vi "首页.vi"() -> ()   [LabVIEW 2016]
uses:
  <vilib>/Utility/miscctls.llb/LVPointTypeDef.ctl
  <vilib>/Utility/sysdir.llb/System Directory Type.ctl
  <vilib>/addons/database/_DB Variant To Data/Database Variant To Data.xnode
  PLC/PLC.lvlib
panel:
  out "大项目框 12":T1(xcontrol)
  out "大项目框 11":T1(xcontrol)
  out "大项目框 10":T1(xcontrol)
  out "大项目框 9":T1(xcontrol)
  out "大项目框 8":T1(xcontrol)
  out "大项目框 7":T1(xcontrol)
  out "大项目框 6":T1(xcontrol)
  out "大项目框 5":T1(xcontrol)
  out "大项目框 4":T1(xcontrol)
  out "大项目框 3":T1(xcontrol)
  out "大项目框 2":T1(xcontrol)
  out "大项目框":T1(xcontrol)
  out "湿度":string="75.5 %"
  out "室温":string="25.8 ℃"
  # "室温:"
  # "湿度:"
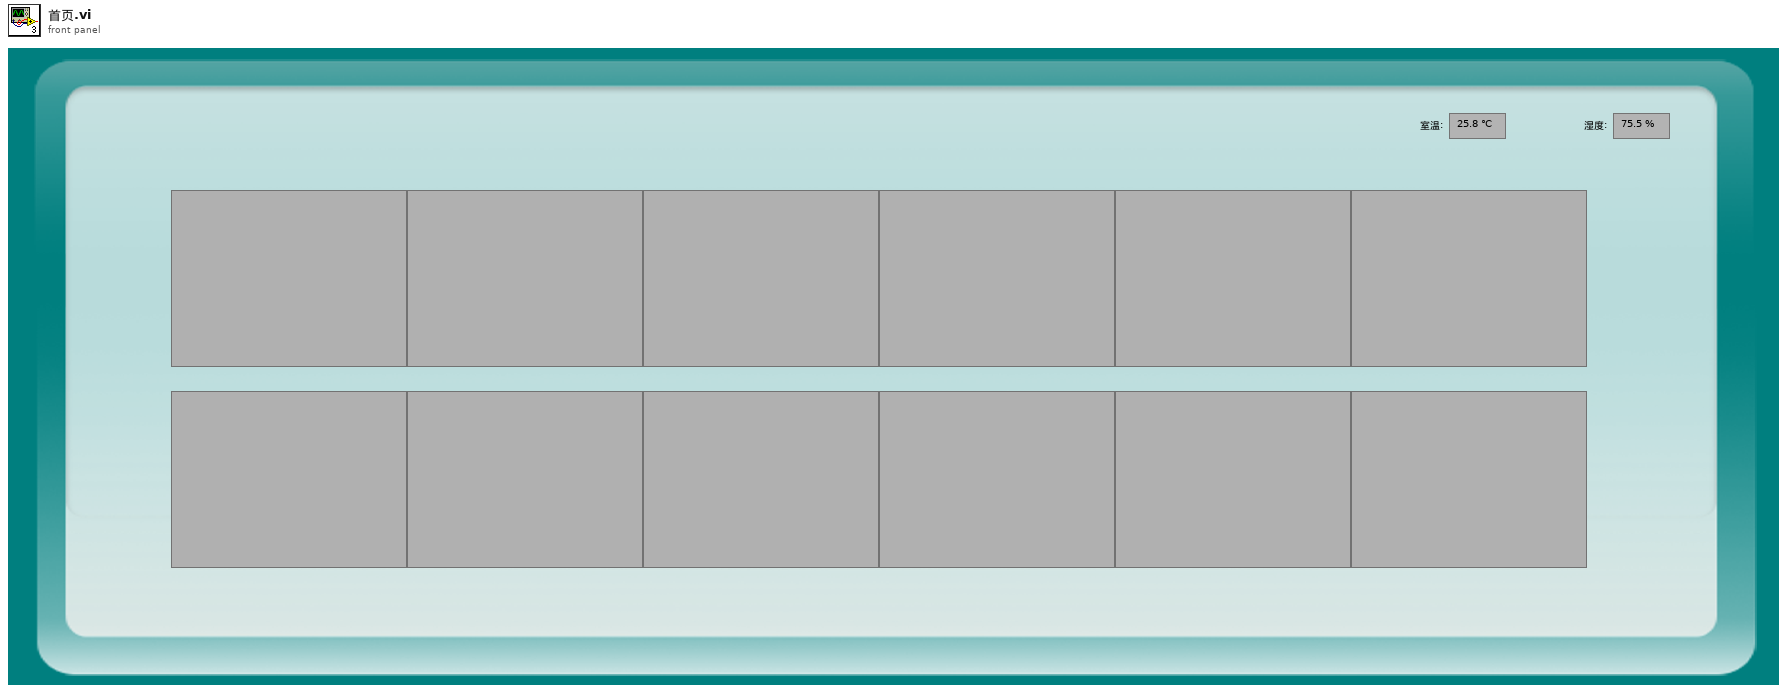
[diagram p1: front panel]
types:
  T1 = cluster{"中文项目名称":string, "英文项目名称":string, "单位":string, "浓度值":string}
  T2 = typedef "LVPointTypeDef.ctl" = cluster{"Horizontal":i16, "Vertical":i16}
  T3 = cluster{"显示参数中文名":string, "显示参数英文名":string, "显示浓度":string, "显示单位":string}[]
  T4 = cluster{"显示参数中文名":string, "显示参数英文名":string, "显示浓度":string, "显示单位":string}
  T5 = typedef "System Directory Type.ctl" = i32
  T6 = cluster{"水温":bool, "pH":bool, "DO":bool, "Cond":bool, "Turb":bool, "氨氮":bool, "总磷":bool, "总氮":bool, "CODMn":bool, "CODCr":bool, "水位":bool, "流速":bool, "瞬时流量":bool, "ORP":bool}
  T7 = cluster{"AD0":sgl, "AD1":sgl, "AD2":sgl, "AD3":sgl, "AD4":sgl, "AD5":sgl}
  T8 = typedef "LVDateTimeRec.ctl" = cluster{"秒数的小数部分":dbl, "秒":i32, "分":i32, "时":i32, "日":i32, "月":i32, "年":i32, "天数（周）":i32, "天数（年）":i32, "DST":i32}
  T9 = cluster{"时间标识":timestamp, "监测值":sgl, "单位":string}
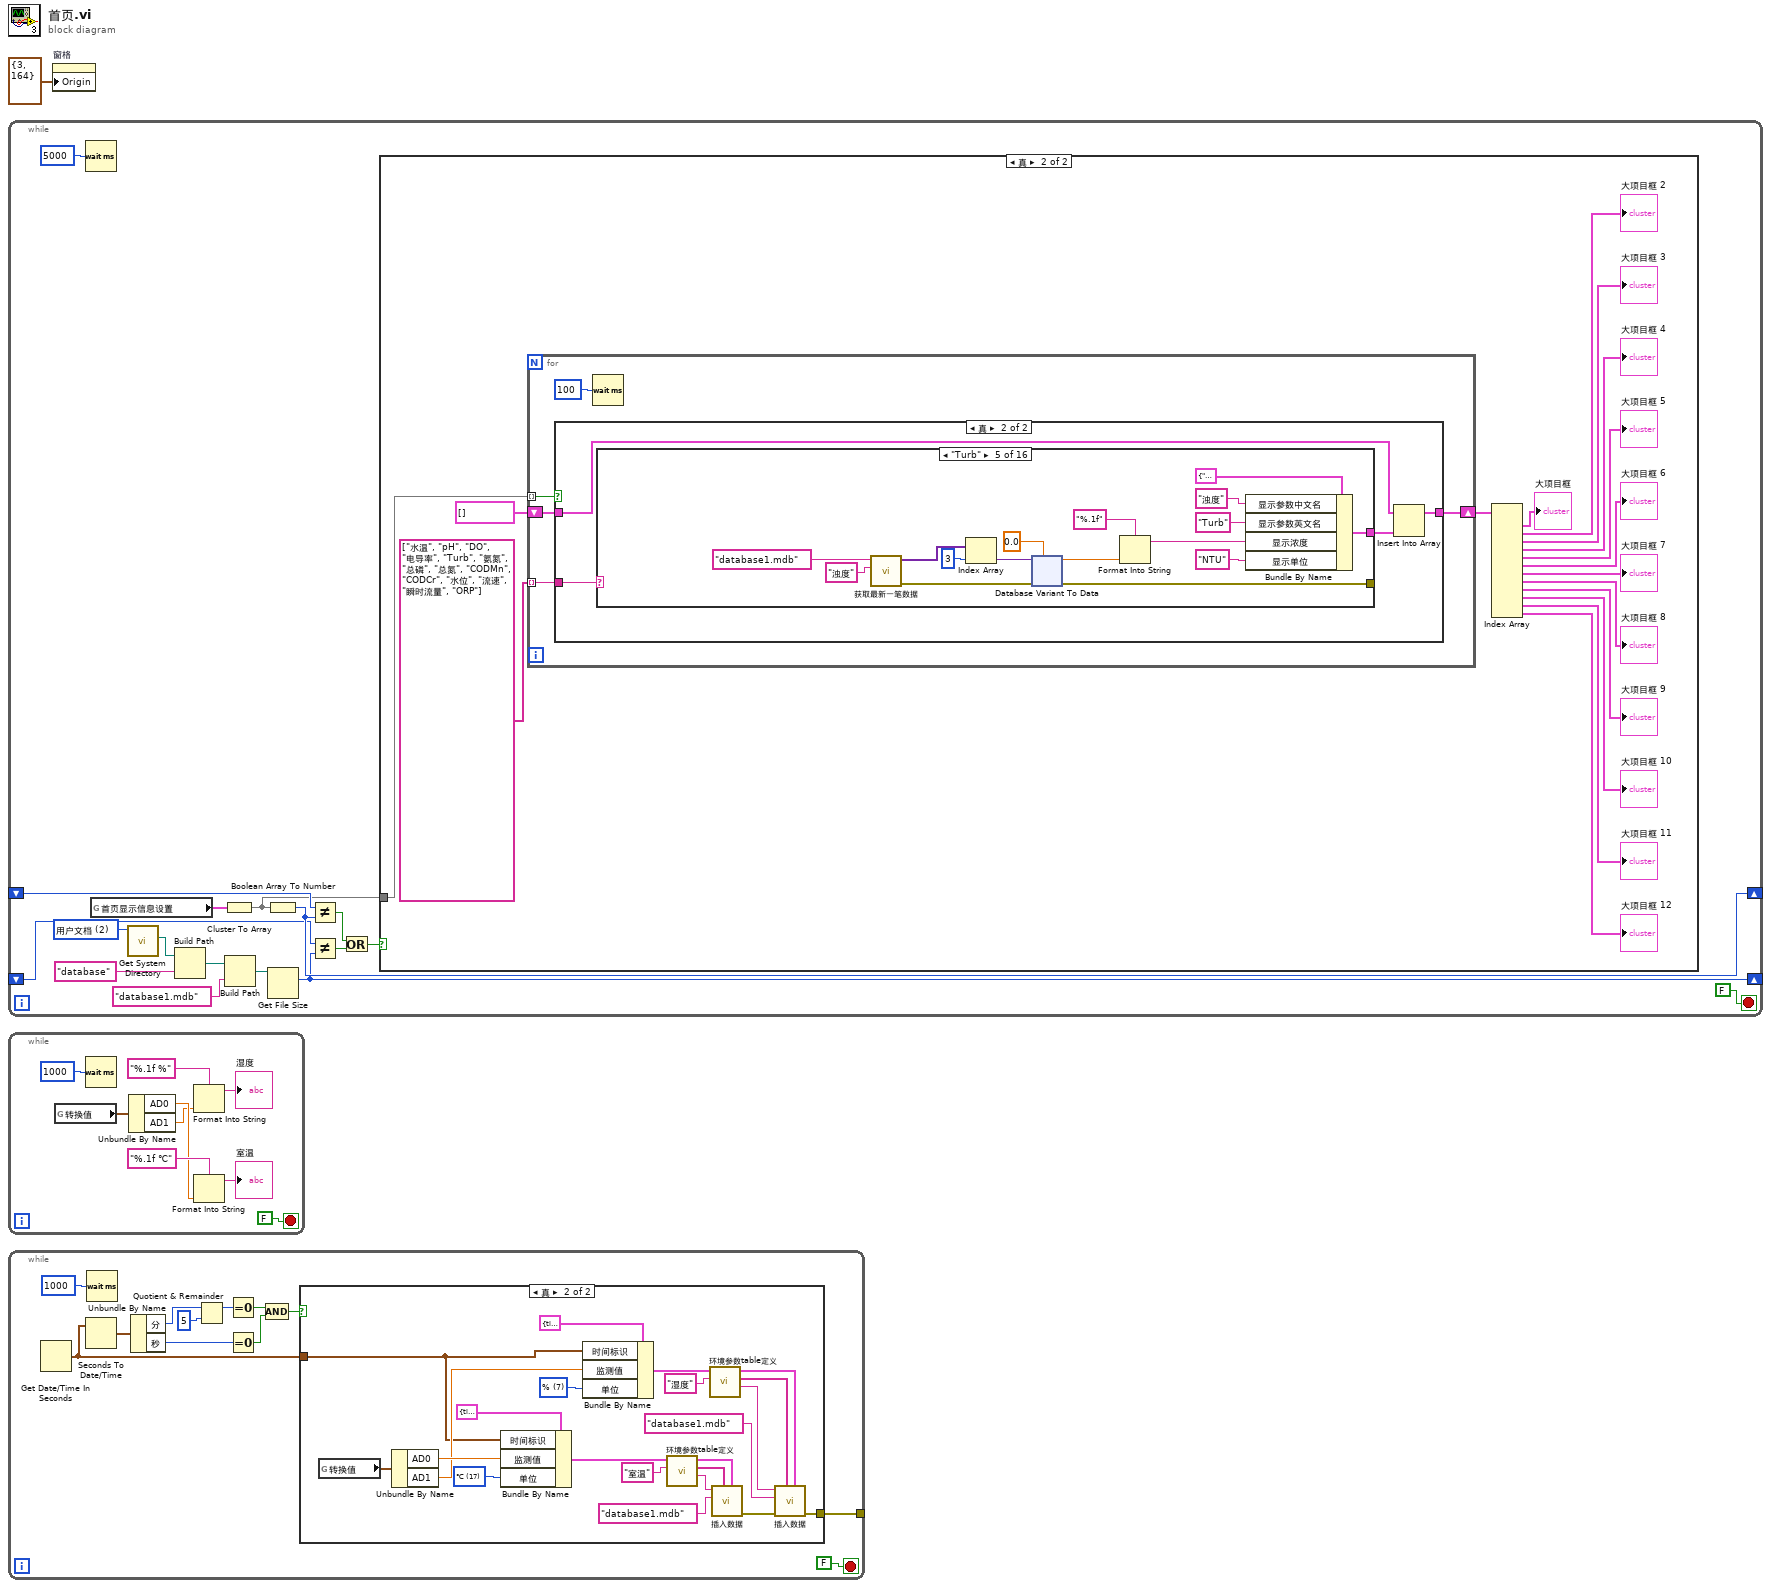
[diagram p0: block diagram]
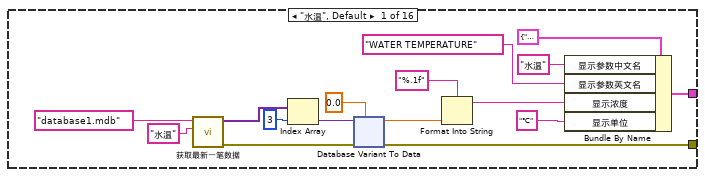
[diagram p5: hidden frame]
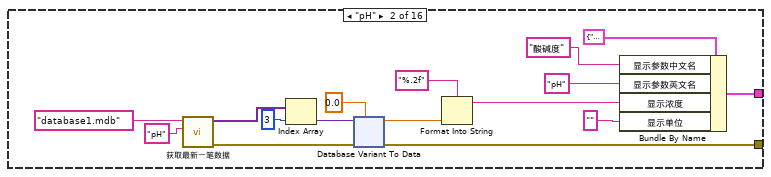
[diagram p6: hidden frame]
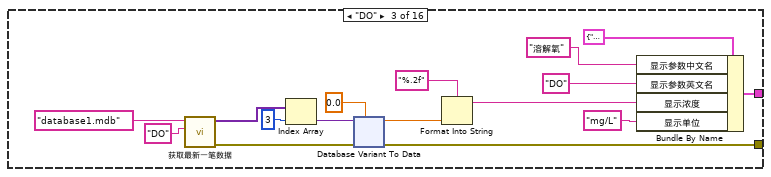
[diagram p7: hidden frame]
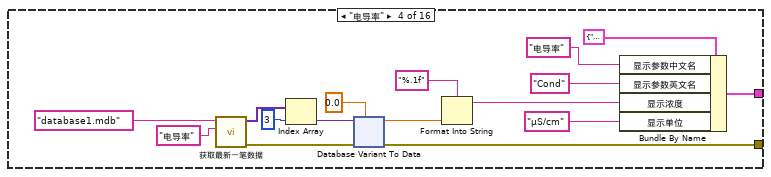
[diagram p8: hidden frame]
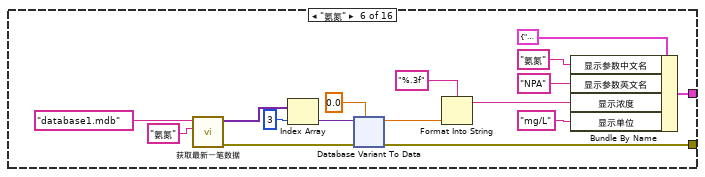
[diagram p9: hidden frame]
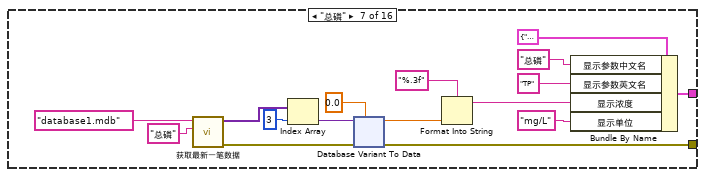
[diagram p10: hidden frame]
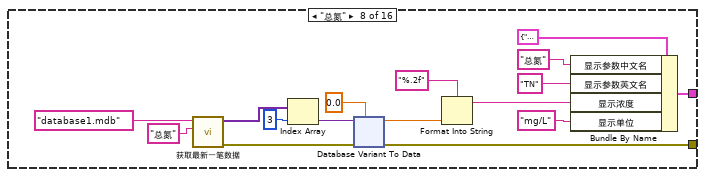
[diagram p11: hidden frame]
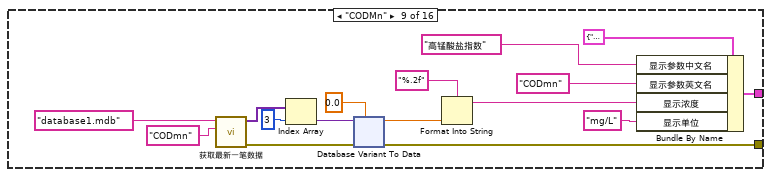
[diagram p12: hidden frame]
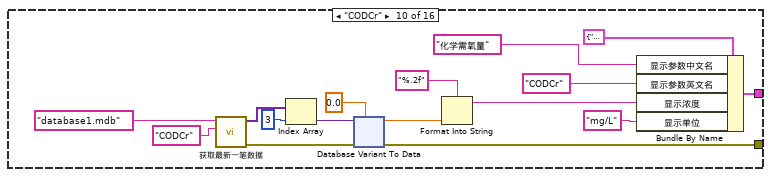
[diagram p13: hidden frame]
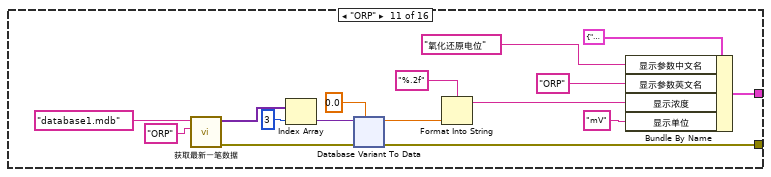
[diagram p14: hidden frame]
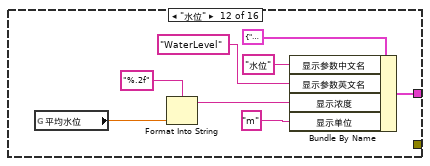
[diagram p15: hidden frame]
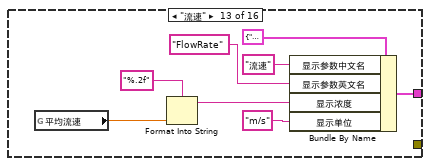
[diagram p16: hidden frame]
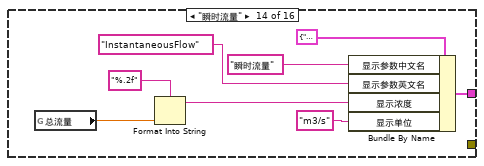
[diagram p17: hidden frame]
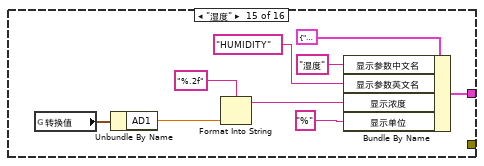
[diagram p18: hidden frame]
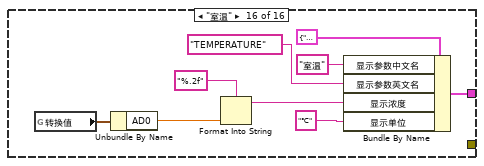
[diagram p19: hidden frame]
diagram:
  n1 = while {
    shift-right: [w13] -> _
    shift-left: _ -> [w15]
    shift-right: [w7] -> _
    shift-left: _ -> [w6]
    stop <- FALSE stop-if-true
    w2 = T5 2 items=["用户目录"=0, "用户桌面"=1, "用户文档"=2, "用户应用程序数据"=3, "用户设置"=4, "用户临时目录"=5, "公共文档"=6, "公共应用程序数据"=7, "公共设置"=8, "公共缓存"=13, "系统核心库"=9, "系统安装库"=10, "应用程序文件"=11, "启动盘根目录"=12] ("system directory type")
    n2 = Wait (ms)(milliseconds to wait=u32 5000 ("等待时间（毫秒）")) -> ()  [unwired: 1 out]
    n3 = global read "系统设置全局变量.vi" "首页显示信息设置"() -> (w16:T6)
    n4 = call <vilib>:"Get System Directory.vi"("system directory type"=w2) -> ("system directory"=w12:path)  [unwired: 10 in]
    n5 = Build Path(base path=w12, name or relative path="database" ("名称或相对路径")) -> (appended path=w10:path)
    n6 = Cluster To Array(cluster=w16) -> (array=w14:bool[])
    n7 = Build Path(base path=w10, name or relative path="database1.mdb" ("名称或相对路径")) -> (appended path=w8:path)
    n8 = Boolean Array To Number(Boolean array=w14) -> (number=w13:u32)
    n9 = Get File Size(file=w8) -> (size (in bytes)=w7:i64)  [unwired: 1 in, 2 out]
    n10 = Not Equal?(x=w15, y=w13) -> (x != y?=w3:bool)
    n11 = Not Equal?(x=w6, y=w7) -> (x != y?=w5:bool)
    n12 = Or(x=w3, y=w5) -> (x .or. y?=w4:bool)
    n13 = case shown="真" w4 {
      tunnel: w14 -> [_ w19]
      frame False {
      }
      frame True {
        n14 = for {
          tunnel: w19 -> [w39] mode=indexing
          tunnel: string[] ["水温", "pH", "DO", "电导率", "Turb", "氨氮", "总磷", "总氮", "CODMn", "CODCr", "水位", "流速", "瞬时流量", "ORP"] -> [w38] mode=indexing
          shift-right: [w36] -> w32
          shift-left: T3 [] -> [w37]
          n15 = case shown="真" w39 {
            tunnel: w38 -> [_ w44]
            tunnel: w37 -> [w40 w43]
            tunnel: [w40 w42] -> w36
            frame False {
            }
            frame True {
              n16 = case shown="\"Turb\"" w44 {
                tunnel: [w45 w104 w152 w200 w248 w296 w344 w392 w440 w488 w536 w576 w584 w589 w601 w610] -> w41
                tunnel: [w46 w93 w141 w189 w237 w285 w333 w381 w429 w477 w525 _ _ _ _ _] -> _
                frame "水温", Default {
                  n17 = call "获取最新一笔数据.vi"("table"="水温", "database"="database1.mdb" ("名称或相对路径")) -> ("error out"=w47:errorcluster, "子数组"=w53:variant[])  [unwired: 8 in]
                  n18 = Index Array(array=w53, index=3 ("索引")) -> (element=w51:variant)
                  n19 = xnode "Database Variant To Data"("database variant"=w51, "error in (no error)"=w47, "type"=0.0) -> ("data"=w48:dbl, "error out"=w46:errorcluster)
                  n20 = Format Into String(format string="%.1f" ("格式字符串"), w48) -> (resulting string=w55:string)  [unwired: 2 in, 1 out]
                  n21 = Bundle By Name(cluster=T4 {"显示参数中文名"="", "显示参数英文名"="", "显示浓度"="", "显示单位"=""} ("元素"), "显示参数中文名"="水温", "显示参数英文名"="WATER TEMPERATURE", "显示浓度"=w55, "显示单位"="℃") -> (w45:T4)
                }
                frame "pH" {
                  n22 = call "获取最新一笔数据.vi"("table"="pH", "database"="database1.mdb" ("名称或相对路径")) -> ("error out"=w94:errorcluster, "子数组"=w100:variant[])  [unwired: 8 in]
                  n23 = Index Array(array=w100, index=3 ("索引")) -> (element=w98:variant)
                  n24 = xnode "Database Variant To Data"("database variant"=w98, "error in (no error)"=w94, "type"=0.0) -> ("data"=w95:dbl, "error out"=w93:errorcluster)
                  n25 = Format Into String(format string="%.2f" ("格式字符串"), w95) -> (resulting string=w102:string)  [unwired: 2 in, 1 out]
                  n26 = Bundle By Name(cluster=T4 {"显示参数中文名"="", "显示参数英文名"="", "显示浓度"="", "显示单位"=""} ("元素"), "显示参数中文名"="酸碱度", "显示参数英文名"="pH", "显示浓度"=w102, "显示单位"="") -> (w104:T4)
                }
                frame "DO" {
                  n27 = call "获取最新一笔数据.vi"("table"="DO", "database"="database1.mdb" ("名称或相对路径")) -> ("error out"=w142:errorcluster, "子数组"=w148:variant[])  [unwired: 8 in]
                  n28 = Index Array(array=w148, index=3 ("索引")) -> (element=w146:variant)
                  n29 = xnode "Database Variant To Data"("database variant"=w146, "error in (no error)"=w142, "type"=0.0) -> ("data"=w143:dbl, "error out"=w141:errorcluster)
                  n30 = Format Into String(format string="%.2f" ("格式字符串"), w143) -> (resulting string=w150:string)  [unwired: 2 in, 1 out]
                  n31 = Bundle By Name(cluster=T4 {"显示参数中文名"="", "显示参数英文名"="", "显示浓度"="", "显示单位"=""} ("元素"), "显示参数中文名"="溶解氧", "显示参数英文名"="DO", "显示浓度"=w150, "显示单位"="mg/L") -> (w152:T4)
                }
                frame "电导率" {
                  n32 = call "获取最新一笔数据.vi"("table"="电导率", "database"="database1.mdb" ("名称或相对路径")) -> ("error out"=w190:errorcluster, "子数组"=w196:variant[])  [unwired: 8 in]
                  n33 = Index Array(array=w196, index=3 ("索引")) -> (element=w194:variant)
                  n34 = xnode "Database Variant To Data"("database variant"=w194, "error in (no error)"=w190, "type"=0.0) -> ("data"=w191:dbl, "error out"=w189:errorcluster)
                  n35 = Format Into String(format string="%.1f" ("格式字符串"), w191) -> (resulting string=w198:string)  [unwired: 2 in, 1 out]
                  n36 = Bundle By Name(cluster=T4 {"显示参数中文名"="", "显示参数英文名"="", "显示浓度"="", "显示单位"=""} ("元素"), "显示参数中文名"="电导率", "显示参数英文名"="Cond", "显示浓度"=w198, "显示单位"="μS/cm") -> (w200:T4)
                }
                frame "Turb" {
                  n37 = call "获取最新一笔数据.vi"("table"="浊度", "database"="database1.mdb" ("名称或相对路径")) -> ("error out"=w238:errorcluster, "子数组"=w244:variant[])  [unwired: 8 in]
                  n38 = Index Array(array=w244, index=3 ("索引")) -> (element=w242:variant)
                  n39 = xnode "Database Variant To Data"("database variant"=w242, "error in (no error)"=w238, "type"=0.0) -> ("data"=w239:dbl, "error out"=w237:errorcluster)
                  n40 = Format Into String(format string="%.1f" ("格式字符串"), w239) -> (resulting string=w246:string)  [unwired: 2 in, 1 out]
                  n41 = Bundle By Name(cluster=T4 {"显示参数中文名"="", "显示参数英文名"="", "显示浓度"="", "显示单位"=""} ("元素"), "显示参数中文名"="浊度", "显示参数英文名"="Turb", "显示浓度"=w246, "显示单位"="NTU") -> (w248:T4)
                }
                frame "氨氮" {
                  n42 = call "获取最新一笔数据.vi"("table"="氨氮", "database"="database1.mdb" ("名称或相对路径")) -> ("error out"=w286:errorcluster, "子数组"=w292:variant[])  [unwired: 8 in]
                  n43 = Index Array(array=w292, index=3 ("索引")) -> (element=w290:variant)
                  n44 = xnode "Database Variant To Data"("database variant"=w290, "error in (no error)"=w286, "type"=0.0) -> ("data"=w287:dbl, "error out"=w285:errorcluster)
                  n45 = Format Into String(format string="%.3f" ("格式字符串"), w287) -> (resulting string=w294:string)  [unwired: 2 in, 1 out]
                  n46 = Bundle By Name(cluster=T4 {"显示参数中文名"="", "显示参数英文名"="", "显示浓度"="", "显示单位"=""} ("元素"), "显示参数中文名"="氨氮", "显示参数英文名"="NPA", "显示浓度"=w294, "显示单位"="mg/L") -> (w296:T4)
                }
                frame "总磷" {
                  n47 = call "获取最新一笔数据.vi"("table"="总磷", "database"="database1.mdb" ("名称或相对路径")) -> ("error out"=w334:errorcluster, "子数组"=w340:variant[])  [unwired: 8 in]
                  n48 = Index Array(array=w340, index=3 ("索引")) -> (element=w338:variant)
                  n49 = xnode "Database Variant To Data"("database variant"=w338, "error in (no error)"=w334, "type"=0.0) -> ("data"=w335:dbl, "error out"=w333:errorcluster)
                  n50 = Format Into String(format string="%.3f" ("格式字符串"), w335) -> (resulting string=w342:string)  [unwired: 2 in, 1 out]
                  n51 = Bundle By Name(cluster=T4 {"显示参数中文名"="", "显示参数英文名"="", "显示浓度"="", "显示单位"=""} ("元素"), "显示参数中文名"="总磷", "显示参数英文名"="TP", "显示浓度"=w342, "显示单位"="mg/L") -> (w344:T4)
                }
                frame "总氮" {
                  n52 = call "获取最新一笔数据.vi"("table"="总氮", "database"="database1.mdb" ("名称或相对路径")) -> ("error out"=w382:errorcluster, "子数组"=w388:variant[])  [unwired: 8 in]
                  n53 = Index Array(array=w388, index=3 ("索引")) -> (element=w386:variant)
                  n54 = xnode "Database Variant To Data"("database variant"=w386, "error in (no error)"=w382, "type"=0.0) -> ("data"=w383:dbl, "error out"=w381:errorcluster)
                  n55 = Format Into String(format string="%.2f" ("格式字符串"), w383) -> (resulting string=w390:string)  [unwired: 2 in, 1 out]
                  n56 = Bundle By Name(cluster=T4 {"显示参数中文名"="", "显示参数英文名"="", "显示浓度"="", "显示单位"=""} ("元素"), "显示参数中文名"="总氮", "显示参数英文名"="TN", "显示浓度"=w390, "显示单位"="mg/L") -> (w392:T4)
                }
                frame "CODMn" {
                  n57 = call "获取最新一笔数据.vi"("table"="CODmn", "database"="database1.mdb" ("名称或相对路径")) -> ("error out"=w430:errorcluster, "子数组"=w436:variant[])  [unwired: 8 in]
                  n58 = Index Array(array=w436, index=3 ("索引")) -> (element=w434:variant)
                  n59 = xnode "Database Variant To Data"("database variant"=w434, "error in (no error)"=w430, "type"=0.0) -> ("data"=w431:dbl, "error out"=w429:errorcluster)
                  n60 = Format Into String(format string="%.2f" ("格式字符串"), w431) -> (resulting string=w438:string)  [unwired: 2 in, 1 out]
                  n61 = Bundle By Name(cluster=T4 {"显示参数中文名"="", "显示参数英文名"="", "显示浓度"="", "显示单位"=""} ("元素"), "显示参数中文名"="高锰酸盐指数", "显示参数英文名"="CODmn", "显示浓度"=w438, "显示单位"="mg/L") -> (w440:T4)
                }
                frame "CODCr" {
                  n62 = call "获取最新一笔数据.vi"("table"="CODCr", "database"="database1.mdb" ("名称或相对路径")) -> ("error out"=w478:errorcluster, "子数组"=w484:variant[])  [unwired: 8 in]
                  n63 = Index Array(array=w484, index=3 ("索引")) -> (element=w482:variant)
                  n64 = xnode "Database Variant To Data"("database variant"=w482, "error in (no error)"=w478, "type"=0.0) -> ("data"=w479:dbl, "error out"=w477:errorcluster)
                  n65 = Format Into String(format string="%.2f" ("格式字符串"), w479) -> (resulting string=w486:string)  [unwired: 2 in, 1 out]
                  n66 = Bundle By Name(cluster=T4 {"显示参数中文名"="", "显示参数英文名"="", "显示浓度"="", "显示单位"=""} ("元素"), "显示参数中文名"="化学需氧量", "显示参数英文名"="CODCr", "显示浓度"=w486, "显示单位"="mg/L") -> (w488:T4)
                }
                frame "ORP" {
                  n67 = call "获取最新一笔数据.vi"("table"="ORP", "database"="database1.mdb" ("名称或相对路径")) -> ("error out"=w526:errorcluster, "子数组"=w532:variant[])  [unwired: 8 in]
                  n68 = Index Array(array=w532, index=3 ("索引")) -> (element=w530:variant)
                  n69 = xnode "Database Variant To Data"("database variant"=w530, "error in (no error)"=w526, "type"=0.0) -> ("data"=w527:dbl, "error out"=w525:errorcluster)
                  n70 = Format Into String(format string="%.2f" ("格式字符串"), w527) -> (resulting string=w534:string)  [unwired: 2 in, 1 out]
                  n71 = Bundle By Name(cluster=T4 {"显示参数中文名"="", "显示参数英文名"="", "显示浓度"="", "显示单位"=""} ("元素"), "显示参数中文名"="氧化还原电位", "显示参数英文名"="ORP", "显示浓度"=w534, "显示单位"="mV") -> (w536:T4)
                }
                frame "水位" {
                  n72 = global read "流量计全局变量.vi" "平均水位"() -> (w573:dbl)
                  n73 = Format Into String(format string="%.2f" ("格式字符串"), w573) -> (resulting string=w574:string)  [unwired: 2 in, 1 out]
                  n74 = Bundle By Name(cluster=T4 {"显示参数中文名"="", "显示参数英文名"="", "显示浓度"="", "显示单位"=""} ("元素"), "显示参数中文名"="水位", "显示参数英文名"="WaterLevel", "显示浓度"=w574, "显示单位"="m") -> (w576:T4)
                }
                frame "流速" {
                  n75 = global read "流量计全局变量.vi" "平均流速"() -> (w581:dbl)
                  n76 = Format Into String(format string="%.2f" ("格式字符串"), w581) -> (resulting string=w582:string)  [unwired: 2 in, 1 out]
                  n77 = Bundle By Name(cluster=T4 {"显示参数中文名"="", "显示参数英文名"="", "显示浓度"="", "显示单位"=""} ("元素"), "显示参数中文名"="流速", "显示参数英文名"="FlowRate", "显示浓度"=w582, "显示单位"="m/s") -> (w584:T4)
                }
                frame "瞬时流量" {
                  n78 = global read "流量计全局变量.vi" "总流量"() -> (w590:dbl)
                  n79 = Format Into String(format string="%.2f" ("格式字符串"), w590) -> (resulting string=w591:string)  [unwired: 2 in, 1 out]
                  n80 = Bundle By Name(cluster=T4 {"显示参数中文名"="", "显示参数英文名"="", "显示浓度"="", "显示单位"=""} ("元素"), "显示参数中文名"="瞬时流量", "显示参数英文名"="InstantaneousFlow", "显示浓度"=w591, "显示单位"="m3/s") -> (w589:T4)
                }
                frame "湿度" {
                  n81 = global read "采配水全局变量.vi" "转换值"() -> (w598:T7)
                  n82 = Unbundle By Name(w598) -> ("AD1"=w600:sgl)
                  n83 = Format Into String(format string="%.2f" ("格式字符串"), w600) -> (resulting string=w597:string)  [unwired: 2 in, 1 out]
                  n84 = Bundle By Name(cluster=T4 {"显示参数中文名"="", "显示参数英文名"="", "显示浓度"="", "显示单位"=""} ("元素"), "显示参数中文名"="湿度", "显示参数英文名"="HUMIDITY", "显示浓度"=w597, "显示单位"="%") -> (w601:T4)
                }
                frame "室温" {
                  n85 = global read "采配水全局变量.vi" "转换值"() -> (w607:T7)
                  n86 = Unbundle By Name(w607) -> ("AD0"=w609:sgl)
                  n87 = Format Into String(format string="%.2f" ("格式字符串"), w609) -> (resulting string=w606:string)  [unwired: 2 in, 1 out]
                  n88 = Bundle By Name(cluster=T4 {"显示参数中文名"="", "显示参数英文名"="", "显示浓度"="", "显示单位"=""} ("元素"), "显示参数中文名"="室温", "显示参数英文名"="TEMPERATURE", "显示浓度"=w606, "显示单位"="℃") -> (w610:T4)
                }
              }
              n89 = Insert Into Array(array=w43, new element=w41) -> (w42:T3)  [unwired: 1 in]
            }
          }
          n90 = Wait (ms)(milliseconds to wait=u32 100 ("等待时间（毫秒）")) -> ()  [unwired: 1 out]
        }
        n91 = Index Array(array=w32) -> (element #1=→"大项目框":T4, element #2=→"大项目框 2":T4, element #3=→"大项目框 3":T4, element #4=→"大项目框 4":T4, element #5=→"大项目框 5":T4, element #6=→"大项目框 6":T4, element #7=→"大项目框 7":T4, element #8=→"大项目框 8":T4, element #9=→"大项目框 9":T4, element #10=→"大项目框 10":T4, element #11=→"大项目框 11":T4, element #12=→"大项目框 12":T4)  [unwired: 12 in]
      }
    }
  }
  n92 = while {
    stop <- FALSE stop-if-true
    n93 = global read "采配水全局变量.vi" "转换值"() -> (w621:T7)
    n94 = Wait (ms)(milliseconds to wait=u32 1000 ("等待时间（毫秒）")) -> ()  [unwired: 1 out]
    n95 = Unbundle By Name(w621) -> ("AD0"=w616:sgl, "AD1"=w615:sgl)
    n96 = Format Into String(format string="%.1f %" ("格式字符串"), w615) -> (resulting string=→"湿度":string)  [unwired: 2 in, 1 out]
    n97 = Format Into String(format string="%.1f ℃" ("格式字符串"), w616) -> (resulting string=→"室温":string)  [unwired: 2 in, 1 out]
  }
  n98 = while {
    tunnel: [w634] -> _
    stop <- FALSE stop-if-true
    n99 = Get Date/Time In Seconds() -> (seconds since 1Jan1904=w633:timestamp)
    n100 = Seconds To Date/Time(time stamp (now)=w633) -> (date time rec=w632:T8)  [unwired: 1 in]
    n101 = Wait (ms)(milliseconds to wait=u32 1000 ("等待时间（毫秒）")) -> ()  [unwired: 1 out]
    n102 = Unbundle By Name(w632) -> ("分"=w631:i32, "秒"=w629:i32)
    n103 = Quotient & Remainder(x=w631, y=5) -> (x-y*floor(x/y)=w628:i32)  [unwired: 1 out]
    n104 = Equal To 0?(x=w628) -> (x = 0?=w627:bool)
    n105 = Equal To 0?(x=w629) -> (x = 0?=w626:bool)
    n106 = Compound Arithmetic op=AND ("复合运算")(w627, w626) -> (w625:bool)
    n107 = case shown="真" w625 {
      tunnel: [_ w649] -> w634
      tunnel: w633 -> [_ w637]
      frame False {
      }
      frame True {
        w642 = u16 7 items=["ug/L", "mg/L", "ppm", "mg/m3", "cm", "ppb", "ug/m3", "%", "nmol/mol", "umol/mol", "MPN/L", "MPN/100ml", "ng/m3", "NTU", "无量纲", "ms/cm", "us/cm", "℃", "V"] ("单位")
        w646 = u16 17 items=["ug/L", "mg/L", "ppm", "mg/m3", "cm", "ppb", "ug/m3", "%", "nmol/mol", "umol/mol", "MPN/L", "MPN/100ml", "ng/m3", "NTU", "无量纲", "ms/cm", "us/cm", "℃", "V"] ("单位")
        n108 = global read "采配水全局变量.vi" "转换值"() -> (w657:T7)
        n109 = Unbundle By Name(w657) -> ("AD0"=w645:sgl, "AD1"=w643:sgl)
        n110 = Bundle By Name(cluster=cluster{"时间标识":timestamp, "监测值":sgl, "单位":u16} {"时间标识"=timestamp(0 s since 1904-01-01), "监测值"=0.0, "单位"=0} ("data"), "时间标识"=w637, "监测值"=w645, "单位"=w646) -> (w647:cluster{"时间标识":timestamp, "监测值":sgl, "单位":u16})
        n111 = Bundle By Name(cluster=cluster{"时间标识":timestamp, "监测值":sgl, "单位":u16} {"时间标识"=timestamp(0 s since 1904-01-01), "监测值"=0.0, "单位"=0} ("data"), "时间标识"=w637, "监测值"=w643, "单位"=w642) -> (w641:cluster{"时间标识":timestamp, "监测值":sgl, "单位":u16})
        n112 = call "环境参数table定义.vi"("table 输入"="室温", "data"=w647) -> ("table 输出"=w656:string, "columns"=w655:string[], "data输出"=w654:T9)  [unwired: 7 in]
        n113 = call "环境参数table定义.vi"("table 输入"="湿度", "data"=w641) -> ("table 输出"=w651:string, "columns"=w652:string[], "data输出"=w653:T9)  [unwired: 7 in]
        n114 = call "插入数据.vi"("data"=w654, "columns"=w655, "database"="database1.mdb" ("table 输入"), "table"=w656) -> ("error out"=w650:errorcluster)  [unwired: 7 in]
        n115 = call "插入数据.vi"("data"=w653, "columns"=w652, "error in (no error)"=w650, "database"="database1.mdb" ("table 输入"), "table"=w651) -> ("error out"=w649:errorcluster)  [unwired: 6 in]
      }
    }
  }
  n116 = property on="窗格" class="Pane"("Origin"=T2 {"Horizontal"=3, "Vertical"=164} ("原点")) -> ()  [unwired: 2 in, 2 out]
